vi "find variables  names by reg exp.vi"(9 "ignore case":bool, 10 "exclude string (reg exp)":string, 11 "search string (reg exp)":string) -> (2 "Array of Variable Names":string[](array[string]), 3 "CRLF delimited string of Variable Names":string)   [LabVIEW 2012]
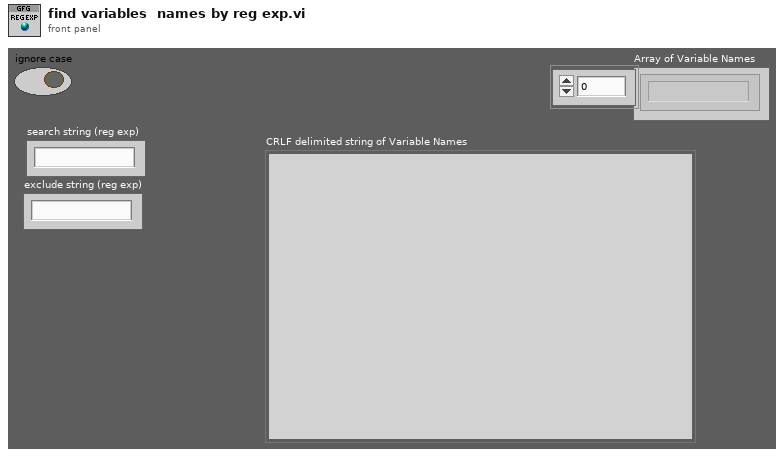
[diagram p1: front panel]
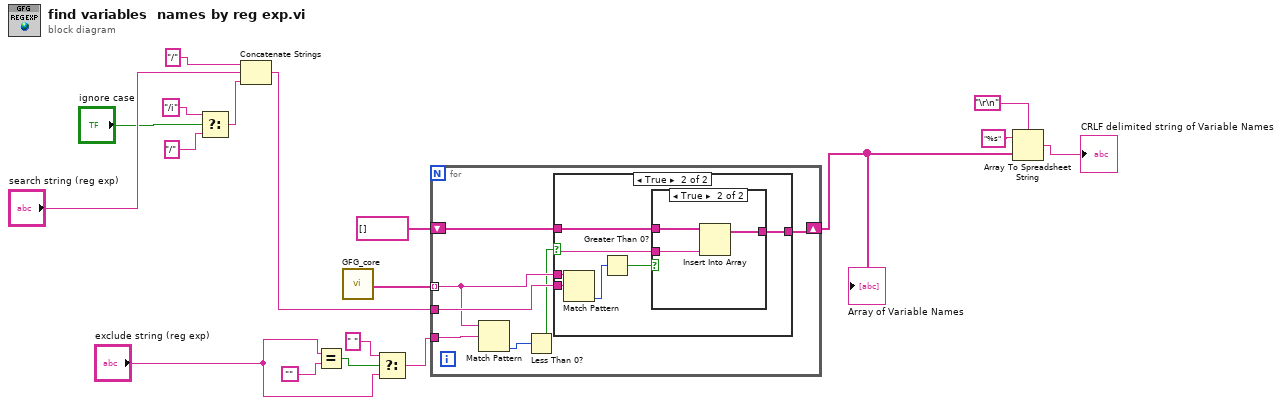
[diagram p0: block diagram]
diagram:
  n1 = Select(t="/i" ("search string (reg exp)"), s="ignore case", f="/" ("search string (reg exp)")) -> (s? t:f=w3:string)
  n2 = Concatenate Strings("/" ("search string (reg exp)"), "search string (reg exp)", w3) -> (w2:string)
  n3 = Equal?(x="exclude string (reg exp)", y="") -> (x = y?=w11:bool)
  n4 = call "GFG_core.vi"() -> ("All Variable Names Out"=w18:string[])  [unwired: 13 in, 6 out]
  n5 = Select(t=" ", s=w11, f="exclude string (reg exp)") -> (s? t:f=w8:string)
  n6 = for {
    tunnel: w18 -> [w21] mode=indexing
    shift-right: [w24] -> w14
    shift-left: string[] [] ("All Variable Names Out") -> [w25]
    tunnel: w2 -> [w23]
    tunnel: w8 -> [w22]
    n7 = Match Pattern(string=w21, regular expression=w22) -> (offset past match=w20:i32)  [unwired: 1 in, 3 out]
    n8 = Less Than 0?(x=w20) -> (x < 0?=w19:bool)
    n9 = case shown="True" w19 {
      tunnel: w25 -> [w26 w31]
      tunnel: [w26 w30] -> w24
      tunnel: w23 -> [_ w28]
      tunnel: w21 -> [_ w27]
      frame False {
      }
      frame True {
        n10 = Match Pattern(string=w27, regular expression=w28) -> (offset past match=w32:i32)  [unwired: 1 in, 3 out]
        n11 = Greater Than 0?(x=w32) -> (x > 0?=w29:bool)
        n12 = case shown="True" w29 {
          tunnel: w31 -> [w33 w36]
          tunnel: [w33 w35] -> w30
          tunnel: w27 -> [_ w34]
          frame False {
          }
          frame True {
            n13 = Insert Into Array(array=w36, new element=w34) -> (w35:string[])  [unwired: 1 in]
          }
        }
      }
    }
  }
  "Array of Variable Names" <- w14
  n14 = Array To Spreadsheet String(delimiter (Tab)="\r\n", array=w14, 3:"%s" ("format string")) -> (spreadsheet string=→"CRLF delimited string of Variable Names":string)
